vi "3458A Setup Virtual Channels.vi"(2 "multiplex cfg":T1={"cycles"=0, "delay [s]"=0.0, "enabled"=FALSE, "overhead [s]"=1.0, "tot smpls"=0, "sub-rec"=0, "overhead [%]"=0.0}, 4 "LEVEL trigger":T2 caption="Cluster", 5 "sample period [s] (1 ms)":dbl=0.001 format="%#_6p", 6 "TRIG source (AUTO)":T3, 7 "apperture [s] (1.4 us)":dbl=1.4e-06 format="%#_6p", 8 "error in":errorcluster, 9 "samples count (100)":i32=100, 10 "voltage ranges [Vpk] (empty: use global default)":dbl[](array[numeric]), 11 "digitizer in":T4={"channels"=[], "sync unit"={"VISA"="", "type"=enum."Picotest U6200A"}, "awg unit"={"type"=enum."Agilent 331xxA to 332xxA", "VISA"="", "enable 10MHz ref"=FALSE, "cmi ckd2"={"VISA"="", "clock source"=enum."Auto", "manual ref clk"=FALSE, "ref clock [Hz]"=0.0}}, "sync mode"=enum."MASTER-SLAVE, MASTER clocked by TIMER", "streaming mode"=FALSE, "idn mode"=enum."Auto", "sampling mode"=enum."DCV", "Ts [s]"=0.0, "sample memory [B]"=0, "proc setup"={"channel id"=0, "packet size [smpl]"=0, "current timeout [s]"=0.0, "blk2blk timeout [s]"=0.0, "event time"=timestamp(0 s since 1904-01-01), "stop notifier"=refnum, "data queues"=[], "proc refs"=[], "bus semaphore"=refnum}, "sample size [B]"=0, "sample count"=0, "aux data"={"channel id"=0, "valid?"=[], "gain [V]"=[], "timestamp [s]"=[], "Ts [s]"=0.0, "abs timestamp"=timestamp(0 s since 1904-01-01), "t [deg C]"=[], "multiplex timestamp [s]"=-1.0, "only multiplex?"=FALSE, "multiplex smpl offset"=0, "overflow?"=FALSE}, "ranges [V]"=[], "aperture [s]"=0.0, "LEVEL trigger"={"edge"=enum."POS", "level [V]"=0.0, "coupling"=enum."DC"}, "trigger mode"=enum."AUTO", "measure temp.?"=FALSE, "disp mesages"=[], "shared bus?"=FALSE, "disable display?"=FALSE, "aper mode"=enum."Manual", "aper rules"=[], "multiplex"={"cycles"=0, "delay [s]"=0.0, "enabled"=FALSE, "overhead [s]"=1.0, "tot smpls"=0, "sub-rec"=0, "overhead [%]"=0.0}, "F8588 lpf"=enum."Off", "F8588 pll"=enum."Off", "F8588 couple"=enum."DC, auto"} {"channels"."Range [Vpk]" min=0.0}) -> (0 "error out":errorcluster, 3 "digitizer out":T4={"channels"=[], "sync unit"={"VISA"="", "type"=enum."Picotest U6200A"}, "awg unit"={"type"=enum."Agilent 331xxA to 332xxA", "VISA"="", "enable 10MHz ref"=FALSE, "cmi ckd2"={"VISA"="", "clock source"=enum."Auto", "manual ref clk"=FALSE, "ref clock [Hz]"=0.0}}, "sync mode"=enum."MASTER-SLAVE, MASTER clocked by TIMER", "streaming mode"=FALSE, "idn mode"=enum."Auto", "sampling mode"=enum."DCV", "Ts [s]"=0.0, "sample memory [B]"=0, "proc setup"={"channel id"=0, "packet size [smpl]"=0, "current timeout [s]"=0.0, "blk2blk timeout [s]"=0.0, "event time"=timestamp(0 s since 1904-01-01), "stop notifier"=refnum, "data queues"=[], "proc refs"=[], "bus semaphore"=refnum}, "sample size [B]"=0, "sample count"=0, "aux data"={"channel id"=0, "valid?"=[], "gain [V]"=[], "timestamp [s]"=[], "Ts [s]"=0.0, "abs timestamp"=timestamp(0 s since 1904-01-01), "t [deg C]"=[], "multiplex timestamp [s]"=-1.0, "only multiplex?"=FALSE, "multiplex smpl offset"=0, "overflow?"=FALSE}, "ranges [V]"=[], "aperture [s]"=0.0, "LEVEL trigger"={"edge"=enum."POS", "level [V]"=0.0, "coupling"=enum."DC"}, "trigger mode"=enum."AUTO", "measure temp.?"=FALSE, "disp mesages"=[], "shared bus?"=FALSE, "disable display?"=FALSE, "aper mode"=enum."Manual", "aper rules"=[], "multiplex"={"cycles"=0, "delay [s]"=0.0, "enabled"=FALSE, "overhead [s]"=1.0, "tot smpls"=0, "sub-rec"=0, "overhead [%]"=0.0}, "F8588 lpf"=enum."Off", "F8588 pll"=enum."Off", "F8588 couple"=enum."DC, auto"} {"channels"."Range [Vpk]" min=0.0})   [LabVIEW 2020, in "3458A Virtual Digitizer.lvlib"]
doc: "This VI setups all channels of a virtual digitizer to desired modes. If vector of ranges is entered it will override default channel settings from the session. It also setups all related instruments to the needed states (AWG and counter). Call this VI at least once before initiating digitizing!"
uses:
  3458A Virtual Digitizer.lvlib
  3458A Digitizer Session.ctl
  3458A Virtual Channel Config.ctl
  Counter/Counter Session.ctl
  Counter/Counter Type.ctl
  AWG/AWG Session.ctl
  AWG/AWG Type.ctl
  AWG/CMI Clock Divider v2/CMI ckd2 Session.ctl
  AWG/CMI Clock Divider v2/CMI ckd2 Source Mode.ctl
  3458A Sync Mode.ctl
  3458A Idn Mode.ctl
  3458A Digitizing Low Levels/Configure/Sampling Mode.ctl
  3458A Digitizing Process Options.ctl
  3458A Data Packet.ctl
  3458A Aux Record Data.ctl
  3458A Digitizing Low Levels/Configure/Level Setup.ctl
  3458A Digitizing Low Levels/Configure/First Sample Trigger.ctl
  3458A Aperture Selection Mode.ctl
  3458A Multiplexing Config.ctl
  Fluke 8588A/F8588A Low Pass Filter.ctl
  Fluke 8588A/F8588A Phase Lock.ctl
  Fluke 8588A/F8588A Coupling.ctl
  3458A Digitizing Low Levels/Configure/EXT OUT mode.ctl
  <vilib>/Utility/error.llb/Error Cluster From Error Code.vi
  <vilib>/ErrorRing/Error Ring.xnode
  3458A Digitizing Low Levels/3458A Digitizing Low Levels.lvlib
  AWG/AWG.lvlib
  Counter/Counter.lvlib
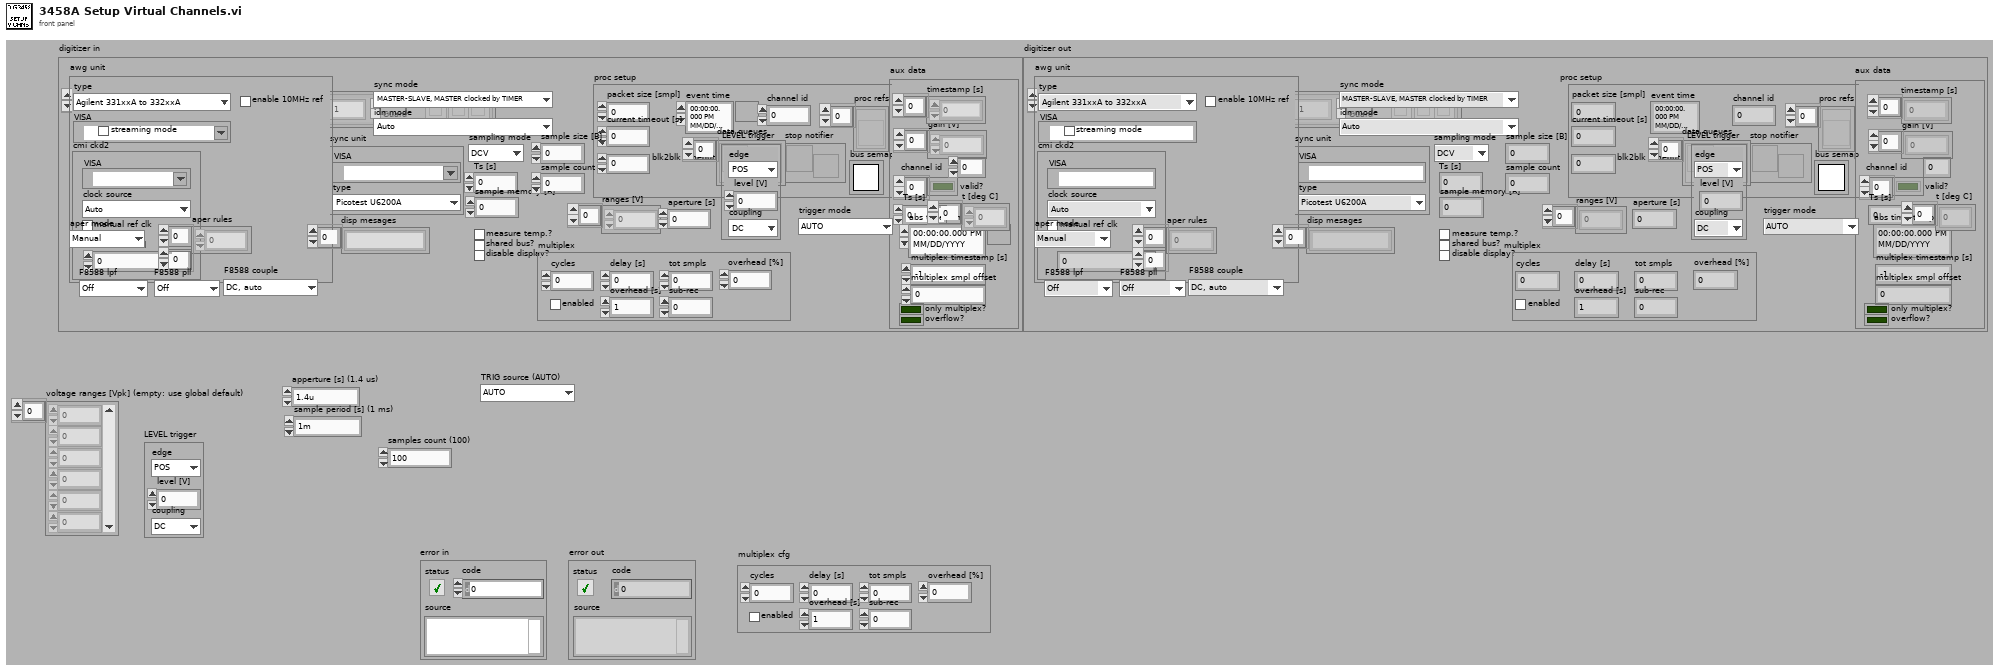
[diagram p1: front panel]
types:
  T1 = typedef "3458A Multiplexing Config.ctl" = cluster{"cycles":i32, "delay [s]":dbl, "enabled":bool, "overhead [s]":dbl, "tot smpls":i64, "sub-rec":i32, "overhead [%]":dbl}
  T2 = typedef "3458A Virtual Digitizer.lvlib/3458A Digitizing Low Levels.lvlib/Level Setup.ctl" = cluster{"edge":enum16{"POS", "NEG"}, "level [V]":dbl, "coupling":enum16{"DC", "AC"}}
  T3 = typedef "3458A Virtual Digitizer.lvlib/3458A Digitizing Low Levels.lvlib/First Sample Trigger.ctl" = enum16{"AUTO", "EXT", "SYN", "SGL", "HOLD", "LEVEL"}
  T4 = typedef "3458A Virtual Digitizer.lvlib/3458A Digitizer Session.ctl" = cluster{"channels":T5[], "sync unit":T6, "awg unit":T8, "sync mode":T12, "streaming mode":bool, "idn mode":T13, "sampling mode":T14, "Ts [s]":dbl, "sample memory [B]":i32, "proc setup":T15, "sample size [B]":i32, "sample count":i32, "aux data":T17, "ranges [V]":dbl[], "aperture [s]":dbl, "LEVEL trigger":T2, "trigger mode":T3, "measure temp.?":bool, "disp mesages":string[], "shared bus?":bool, "disable display?":bool, "aper mode":T18, "aper rules":dbl[][], "multiplex":T1, "F8588 lpf":T19, "F8588 pll":T20, "F8588 couple":T21}
  T5 = typedef "3458A Virtual Digitizer.lvlib/3458A Virtual Channel Config.ctl" = cluster{"VISA":refnum<visa-resource-name>, "Range [Vpk]":dbl, "btn clr":bool, "btn up":bool, "btn down":bool, "F8588":bool, "F8588 guard":bool}
  T6 = typedef "Counter.lvlib/Counter Session.ctl" = cluster{"VISA":refnum<visa-resource-name>, "type":T7}
  T7 = typedef "Counter.lvlib/Counter Type.ctl" = enum16{"Picotest U6200A", "dummy"}
  T8 = typedef "AWG.lvlib/AWG Session.ctl" = cluster{"type":T9, "VISA":refnum<visa-resource-name>, "enable 10MHz ref":bool, "cmi ckd2":T10}
  T9 = typedef "AWG.lvlib/AWG Type.ctl" = enum16{"Agilent 331xxA to 332xxA", "Agilent 335xxA to 336xxA", "Tektronix AFG3101C", "CMI Clock Divider v2", "dummy"}
  T10 = typedef "AWG.lvlib/CMI ckd2 Session.ctl" = cluster{"VISA":refnum<visa-resource-name>, "clock source":T11, "manual ref clk":bool, "ref clock [Hz]":dbl}
  T11 = typedef "AWG.lvlib/CMI ckd2 Source Mode.ctl" = enum16{"Auto", "LF clock", "HF clock", "Internal"}
  T12 = typedef "3458A Virtual Digitizer.lvlib/3458A Sync Mode.ctl" = enum16{"MASTER-SLAVE, MASTER clocked by TIMER", "MASTER-SLAVE, MASTER clocked by AWG", "ALL clocked by AWG", "MASTER-SLAVE, ALL clocked by TIMER", "ALL clocked by AWG with DFLL"}
  T13 = typedef "3458A Virtual Digitizer.lvlib/3458A Idn Mode.ctl" = enum16{"Auto", "Sequential (chn A, chn B, ...)", "From calibration string"}
  T14 = typedef "3458A Virtual Digitizer.lvlib/3458A Digitizing Low Levels.lvlib/Sampling Mode.ctl" = enum16{"DCV", "DSDC", "DSAC"}
  T15 = typedef "3458A Virtual Digitizer.lvlib/3458A Digitizing Process Options.ctl" = cluster{"channel id":i32, "packet size [smpl]":i32, "current timeout [s]":dbl, "blk2blk timeout [s]":dbl, "event time":timestamp, "stop notifier":refnum<notifier>, "data queues":refnum<queue>[], "proc refs":refnum<vi>[], "bus semaphore":T16}
  T16 = typedef "Semaphore RefNum" = refnum<k1>
  T17 = typedef "3458A Virtual Digitizer.lvlib/3458A Aux Record Data.ctl" = cluster{"channel id":i32, "valid?":bool[], "gain [V]":dbl[], "timestamp [s]":dbl[], "Ts [s]":dbl, "abs timestamp":timestamp, "t [deg C]":dbl[], "multiplex timestamp [s]":dbl, "only multiplex?":bool, "multiplex smpl offset":i64, "overflow?":bool}
  T18 = typedef "3458A Virtual Digitizer.lvlib/3458A Aperture Selection Mode.ctl" = enum16{"Manual", "Maximum", "Table"}
  T19 = typedef "F8588A Low Pass Filter.ctl" = enum16{"Off", "100 kHz", "3 MHz"}
  T20 = typedef "F8588A Phase Lock.ctl" = enum16{"Off", "1 MHz", "10 MHz"}
  T21 = typedef "F8588A Coupling.ctl" = enum16{"AC, 1 MOhm", "AC, 10 MOhm", "DC, 1 MOhm", "DC, 10 MOhm", "DC, auto"}
  T22 = typedef "3458A Virtual Digitizer.lvlib/3458A Digitizing Low Levels.lvlib/EXT OUT mode.ctl" = enum16{"APER", "ICOMP"}
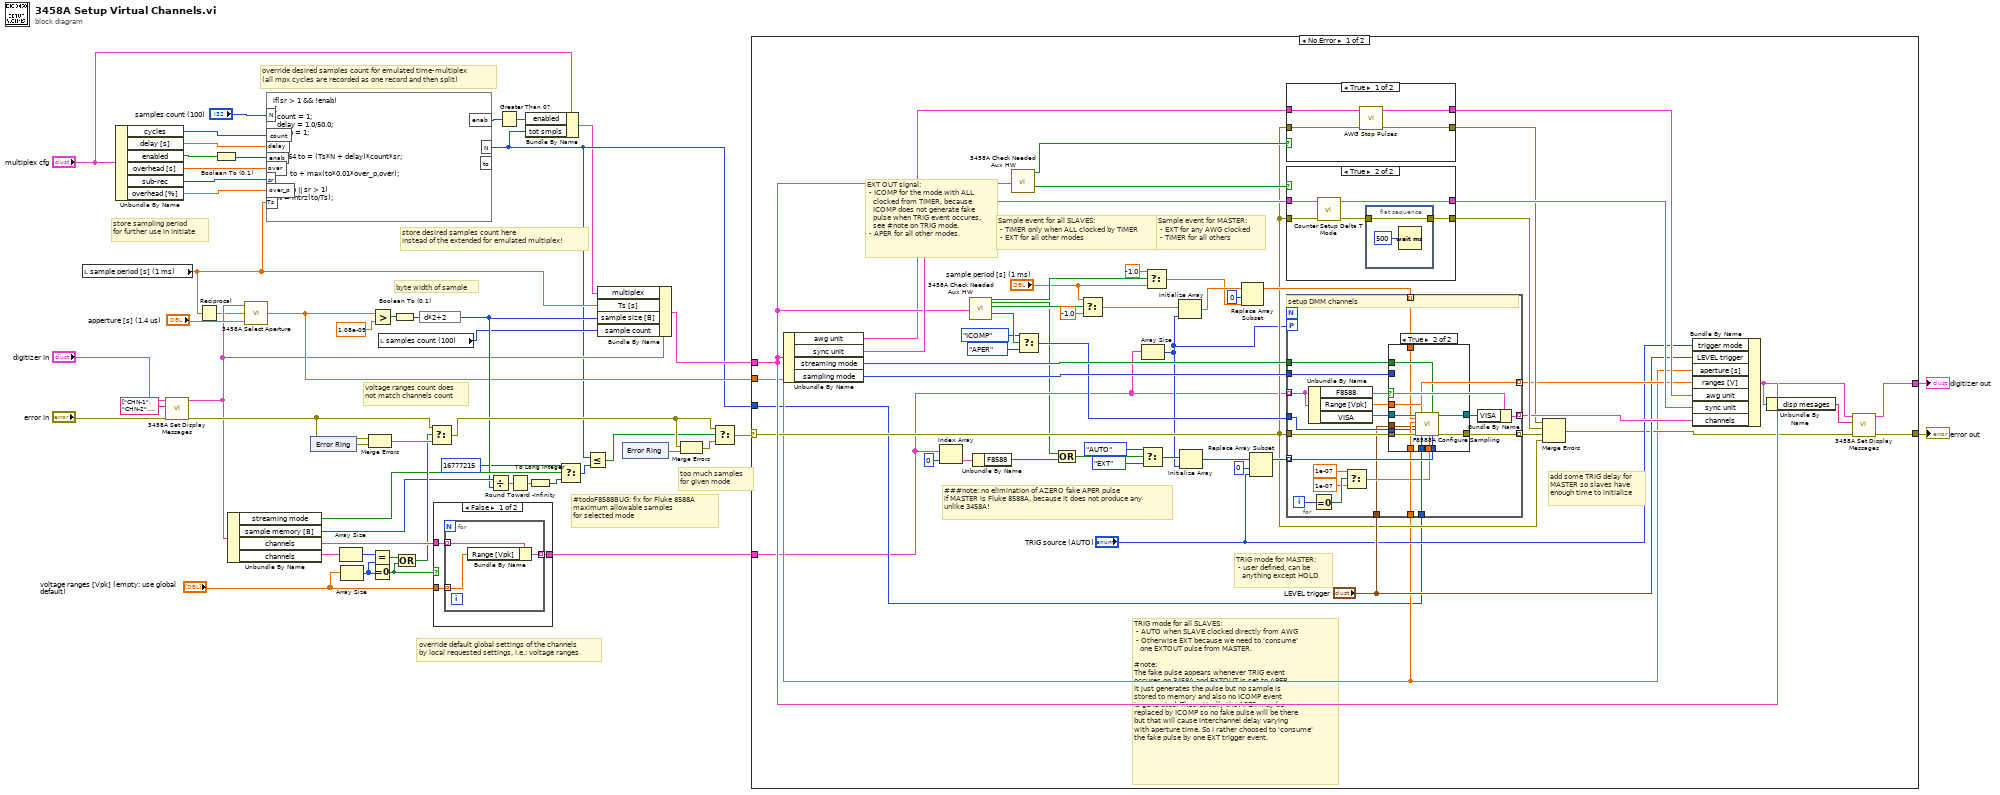
[diagram p0: block diagram]
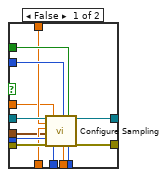
[diagram p4: hidden frame]
diagram:
  # "store desired samples count here\ninstead of the extended for emulated multiplex!"
  # "override desired samples count for emulated time-multiplex\n(all mpx cycles are recorded as one record and then split)"
  # "store sampling period\nfor further use in initiate"
  # "voltage ranges count does\nnot match channels count"
  # "#todoF8588BUG: fix for Fluke 8588A\nmaximum allowable samples\nfor selected mode"
  # "byte width of sample"
  # "too much samples\nfor given mode"
  # "override default global settings of the channels\nby local requested settings, i.e.: voltage ranges"
  n1 = local read "sample period [s] (1 ms)"() -> (w9:dbl)
  n2 = Unbundle By Name("multiplex cfg") -> ("cycles"=w15:i32, "delay [s]"=w13:dbl, "enabled"=w12:bool, "overhead [s]"=w10:dbl, "sub-rec"=w4:i32, "overhead [%]"=w3:dbl)
  n3 = call "3458A Set Display Messages.vi"("error in (no error)"="error in", "display strings"=string[] ["CHN-1", "CHN-2", "CHN-3"], "digitizer session in"="digitizer in") -> ("error out"=w22:errorcluster, "digitizer session out"=w17:T4)  [unwired: 7 in]
  n4 = Reciprocal(x=w9) -> (1/x=w16:dbl)
  n5 = Boolean To (0,1)(Boolean=w12) -> (0, 1=w11:i16)
  n6 = Unbundle By Name(w17) -> ("streaming mode"=w34:bool, "sample memory [B]"=w29:i32, "channels"=w50:T5[], "channels"=w51:T5[])
  n7 = call "3458A Select Aperture.vi"("manual aperture [s]"="apperture [s] (1.4 us)", "sampling rate [Sa/s]"=w16, "digitizer session"=w17) -> ("selected aperture [s]"=w18:dbl)
  n8 = formula code="if(sr > 1 && !enab)\n{\n  count = 1;\n  delay = 1.0/50.0;\n  enab = 1;\n}\n\nfloat64 to = (Ts*N + delay)*count*sr;\n\nto = to + max(to*0.01*over_p,over);\n\nif(enab || sr > 1)\n  N = intrz(to/Ts);"("N"="samples count (100)", "enab"=w11, "delay"=w13, "over"=w10, "count"=w15, "Ts"=w9, "sr"=w4, "over_p"=w3) -> ("N"=w6:i32, "enab"=w2:i16)  [unwired: 1 out]
  n9 = xnode "Error Ring"() -> ("error out"=w49:errorcluster)
  n10 = Array Size(array=w51) -> (size(s)=w39:i32)
  n11 = Array Size(array="voltage ranges [Vpk] (empty: use global default)") -> (size(s)=w43:i32)
  n12 = Merge Errors(w22, w49) -> (w48:errorcluster)
  n13 = Equal?(x=w39, y=w43) -> (x = y?=w44:bool)
  n14 = Equal To 0?(x=w43) -> (x = 0?=w40:bool)
  n15 = Greater?(x=w18, y=1.08e-05) -> (0:w37:bool)
  n16 = local read "samples count (100)"() -> (w7:i32)
  n17 = Boolean To (0,1)(Boolean=w37) -> (0, 1=w36:i16)
  n18 = Compound Arithmetic op=OR(w44, w40) -> (w42:bool)
  n19 = expression code="d*2+2"(w36) -> (w27:i16)
  n20 = Select(t=w22, s=w42, f=w48) -> (s? t:f=w45:errorcluster)
  n21 = case shown="False" w40 {
    tunnel: w50 -> [w56 w60]
    tunnel: [w55 w60] -> w30
    tunnel: "voltage ranges [Vpk] (empty: use global default)" -> [w54 _]
    frame False {
      n22 = for {
        tunnel: w56 -> [w59] mode=indexing
        tunnel: w54 -> [w57] mode=indexing
        tunnel: [w58] -> w55 mode=indexing
        n23 = Bundle By Name(cluster=w59, "Range [Vpk]"=w57) -> (w58:T5)
      }
    }
    frame True {
    }
  }
  n24 = Divide(x=w29, y=w27) -> (x/y=w28:dbl)
  n25 = Greater Than 0?(x=w2) -> (x > 0?=w1:bool)
  n26 = Round Toward -Infinity(1:w28) -> (0:w25:dbl)
  n27 = Bundle By Name(cluster="multiplex cfg", "enabled"=w1, "tot smpls"=w6) -> (w5:T1)
  n28 = To Long Integer(number=w25) -> (32bit integer=w24:i32)
  n29 = Select(t=16777215, s=w34, f=w24) -> (s? t:f=w35:i32)
  n30 = Less Or Equal?(x=w6, y=w35) -> (x <= y?=w33:bool)
  n31 = Bundle By Name(cluster=w17, "multiplex"=w5, "Ts [s]"=w9, "sample size [B]"=w27, "sample count"=w7) -> (w31:T4)
  n32 = xnode "Error Ring"() -> ("error out"=w46:errorcluster)
  n33 = Merge Errors(w45, w46) -> (w47:errorcluster)
  n34 = Select(t=w45, s=w33, f=w47) -> (s? t:f=w32:errorcluster)
  n35 = case shown="No Error" w32 {
    selector: w32 -> [w70 w176]
    tunnel: [w73 w175] -> w53
    tunnel: [w74 w176] -> w52
    tunnel: w31 -> [w91 w175]
    tunnel: w30 -> [w66 _]
    tunnel: w18 -> [w68 _]
    tunnel: w6 -> [w67 _]
    frame No Error {
      # "###note: no elimination of AZERO fake APER pulse\nif MASTER is Fluke 8588A, because it does not produce any\nunlike 3458A!"
      # "EXT OUT signal:\n - ICOMP for the mode with ALL\n   clocked from TIMER, because\n   ICOMP does not generate fake\n   pulse when TRIG event occures,\n   see #note on TRIG mode.\n - APER for all other modes."
      # "add some TRIG delay for\nMASTER so slaves have\nenough time to initialize"
      # "Sample event for MASTER:\n - EXT for any AWG clocked\n - TIMER for all others"
      # "Sample event for all SLAVES:\n - TIMER only when ALL clocked by TIMER\n - EXT for all other modes"
      # "TRIG mode for MASTER:\n - user defined, can be\n   anything except HOLD"
      # "TRIG mode for all SLAVES:\n - AUTO when SLAVE clocked directly from AWG\n - Otherwise EXT because we need to 'consume' \n   one EXTOUT pulse from MASTER.\n\n#note:\nThe fake pulse appears whenever TRIG event \noccures on 3458A and EXTOUT is set to APER.\nIt just generates the pulse but no sample is\nstored to memory and also no ICOMP event\nis generated. Theoretically the APER may be\nreplaced by ICOMP so no fake pulse will be there\nbut that will cause interchannel delay varying\nwith aperture time. So I rather choosed to 'consume'\nthe fake pulse by one EXT trigger event."
      n36 = Unbundle By Name(w91) -> ("awg unit"=w88:T8, "sync unit"=w107:T6, "streaming mode"=w105:bool, "sampling mode"=w104:T14)
      n37 = Index Array(array=w66, index=0) -> (element=w64:T5)
      n38 = call "3458A Check Needed Aux HW.vi"("digitizer session"=w91) -> ("uses AWG clocking?"=w93:bool, "SLAVEs clocked by AWG?"=w63:bool, "SLAVEs clocked from TIMER?"=w85:bool, "uses counter for delta T sync?"=w82:bool)  [unwired: 13 in, 2 out]
      n39 = Unbundle By Name(w64) -> ("F8588"=w61:bool)
      n40 = call "3458A Check Needed Aux HW.vi"("digitizer session"=w91) -> ("uses AWG clocking?"=w89:bool, "uses counter for delta T sync?"=w90:bool)  [unwired: 13 in, 4 out]
      n41 = Select(t=EXT_OUT_mode."ICOMP" ("EXT OUT signal (APER)"), s=w82, f=EXT_OUT_mode."APER" ("EXT OUT signal (APER)")) -> (s? t:f=w79:T22)
      n42 = Compound Arithmetic op=OR(w63, w61) -> (w62:bool)
      n43 = Select(t="sample period [s] (1 ms)", s=w85, f=-1.0 ("t")) -> (s? t:f=w101:dbl)
      n44 = Select(t=First_Sample_Trigger."AUTO" ("first sample (AUTO)"), s=w62, f=First_Sample_Trigger."EXT" ("first sample (AUTO)")) -> (s? t:f=w95:T3)
      n45 = Array Size(array=w66) -> (size(s)=w69:i32)
      n46 = Select(t=-1.0, s=w93, f="sample period [s] (1 ms)") -> (s? t:f=w97:dbl)
      n47 = Initialize Array(w101, w69) -> (w100:dbl[])
      n48 = Initialize Array(w95, w69) -> (w110:T3[])
      n49 = Replace Array Subset(array=w100, new element=w97, index=0) -> (w98:dbl[])
      n50 = Replace Array Subset(array=w110, new element="TRIG source (AUTO)", index=0) -> (w108:T3[])
      n51 = case shown="True" w89 {
        tunnel: w70 -> [w115 w116]
        tunnel: [w113 w116] -> w87
        tunnel: w88 -> [w114 w117]
        tunnel: [w112 w117] -> w86
        frame True {
          # "init AWG for external sample clocking"
          n52 = call "AWG Stop Pulses.vi"("error in (no error)"=w115, "awg session in"=w114) -> ("error out"=w113:errorcluster, "awg session out"=w112:T8)  [unwired: 8 in]
        }
        frame False {
          # "init counter for two DMM delta T\nmeasurement"
        }
      }
      n53 = case shown="True" w90 {
        tunnel: w107 -> [w119 w121]
        tunnel: w70 -> [w118 w123]
        tunnel: [w118 w124] -> w106
        tunnel: [w119 w120] -> w102
        frame False {
        }
        frame True {
          # "init counter for two DMM delta T\nmeasurement"
          n54 = call "Counter Setup Delta T Mode.vi"("error in"=w123, "counter session in"=w121) -> ("error out"=w122:errorcluster, "counter session out"=w120:T6)  [unwired: 8 in]
          n55 = flat-sequence {
            tunnel: [w126] -> w124
            tunnel: w122 -> [w126]
            frame #0 {
              n56 = Wait (ms)(milliseconds to wait=u32 500) -> ()  [unwired: 1 out]
            }
          }
        }
      }
      n57 = for {
        tunnel: w70 -> [w147]
        tunnel: w66 -> [w140] mode=indexing
        tunnel: [w146] -> w111 mode=indexing
        tunnel: [w138] -> w103 mode=indexing
        tunnel: w68 -> [w130]
        tunnel: w67 -> [w143]
        tunnel: w108 -> [w144] mode=indexing
        tunnel: w105 -> [w142]
        tunnel: w104 -> [w141]
        tunnel: w98 -> [w137] mode=indexing
        workers-P: w69 -> [_]
        tunnel: w79 -> [w131]
        tunnel: "LEVEL trigger" -> [w129]
        tunnel: [w128] -> w78 mode=indexing
        i -> [w136]
        # "setup DMM channels"
        n58 = Unbundle By Name(w140) -> ("F8588"=w127:bool, "Range [Vpk]"=w128:dbl, "VISA"=w145:refnum<visa-resource-name>)
        n59 = Equal To 0?(x=w136) -> (x = 0?=w135:bool)
        n60 = Select(t=1e-07, s=w135, f=1e-07) -> (s? t:f=w134:dbl)
        n61 = case shown="True" w127 {
          tunnel: w147 -> [w161 w174]
          tunnel: [w160 w173] -> w146
          tunnel: w145 -> [w159 w171]
          tunnel: w144 -> [w158 w162]
          tunnel: w143 -> [w157 w164]
          tunnel: w142 -> [w156 w170]
          tunnel: w141 -> [w155 _]
          tunnel: [w154 w172] -> w139
          tunnel: w137 -> [w153 w168]
          tunnel: w134 -> [w152 w163]
          tunnel: w131 -> [w151 w165]
          tunnel: w130 -> [w150 w167]
          tunnel: w129 -> [w149 w166]
          tunnel: w128 -> [w148 w169]
          frame False {
            n62 = call "Configure Sampling.vi"("VISA resource in"=w159, "sample period [s] (-1: use EXT trig as source)"=w153, "apperture [s] (1.4us)"=w150, "LEVEL trigger"=w149, "EXT OUT signal (APER)"=w151, "error in"=w161, "range [V] (10V)"=w148, "samples count (100)"=w157, "sampling mode (DCV)"=w155, "delay [s]"=w152, "stream mode (False)"=w156, "first sample (AUTO)"=w158) -> ("VISA resource name out"=w154:refnum<visa-resource-name>, "error out"=w160:errorcluster)  [unwired: 6 in]
          }
          frame True {
            n63 = call "F8588A Configure Sampling.vi"("VISA resource in"=w171, "sample period [s] (-1: use EXT trig as source)"=w168, "apperture [s] (1.4us)"=w167, "LEVEL trigger"=w166, "EXT OUT signal (APER)"=w165, "error in"=w174, "range [V] (10V)"=w169, "samples count (100)"=w164, "delay [s]"=w163, "stream mode (False)"=w170, "first sample (AUTO)"=w162) -> ("VISA resource name out"=w172:refnum<visa-resource-name>, "error out"=w173:errorcluster)  [unwired: 7 in]
          }
        }
        n64 = Bundle By Name(cluster=w140, "VISA"=w139) -> (w138:T5)
      }
      n65 = Merge Errors(w87, w106, w111, w70) -> (w75:errorcluster)
      n66 = Bundle By Name(cluster=w91, "trigger mode"="TRIG source (AUTO)", "LEVEL trigger"="LEVEL trigger", "aperture [s]"=w68, "ranges [V]"=w78, "awg unit"=w86, "sync unit"=w102, "channels"=w103) -> (w72:T4)
      n67 = Unbundle By Name(w72) -> ("disp mesages"=w71:string[])
      n68 = call "3458A Set Display Messages.vi"("error in (no error)"=w75, "display strings"=w71, "digitizer session in"=w72) -> ("error out"=w74:errorcluster, "digitizer session out"=w73:T4)  [unwired: 7 in]
    }
    frame Error {
    }
  }
  "error out" <- w52
  "digitizer out" <- w53
